vi "Wait on CMD Task.vi"(8 "error in (no error)":errorcluster, 9 "Programmer Name":string, 10 "Flash Timeout (ms)":i32=45000, 11 "Slide in":refnum<vi>) -> (0 "error out":errorcluster, 3 "Timed out?":bool)   [LabVIEW 2015]
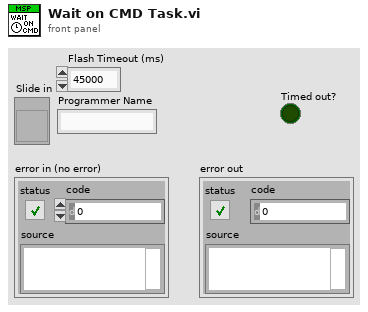
[diagram p1: front panel]
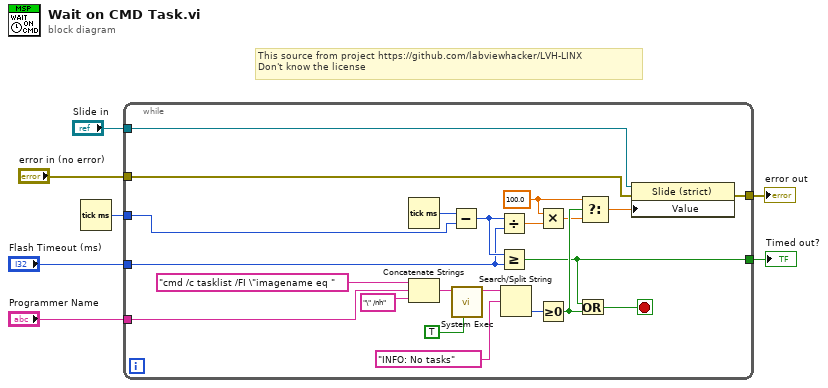
[diagram p0: block diagram]
diagram:
  # "This source from project https://github.com/labviewhacker/LVH-LINX\nDon't know the license"
  n1 = Tick Count (ms)() -> (millisecond timer value=w2:u32)
  n2 = while {
    tunnel: w2 -> [w28]
    tunnel: [w27] -> w4
    tunnel: "error in (no error)" -> [w26]
    tunnel: "Slide in" -> [w25]
    tunnel: [w13] -> w1
    tunnel: "Programmer Name" -> [w9]
    tunnel: "Flash Timeout (ms)" -> [w8]
    stop <- w19 stop-if-true
    w16 = 100.0 ("x")
    n3 = Tick Count (ms)() -> (millisecond timer value=w29:u32)
    n4 = Concatenate Strings("cmd /c tasklist /FI \"imagename eq " ("command line"), w9, "\" /nh" ("string")) -> (w11:string)
    n5 = Subtract(x=w29, y=w28) -> (x-y=w24:u32)
    n6 = call <vilib>:"System Exec.vi"("run minimized? (F)"=TRUE, "command line"=w11) -> ("standard output"=w21:string)  [unwired: 6 in, 3 out]
    n7 = Divide(x=w24, y=w8) -> (x/y=w23:dbl)
    n8 = Greater Or Equal?(x=w24, y=w8) -> (x >= y?=w13:bool)
    n9 = Search/Split String(string=w21, search string/char (-)="INFO: No tasks") -> (offset of match=w18:i32)  [unwired: 1 in, 2 out]
    n10 = Multiply(x=w16, y=w23) -> (x*y=w15:dbl)
    n11 = Greater Or Equal To 0?(x=w18) -> (x >= 0?=w17:bool)
    n12 = Or(x=w13, y=w17) -> (x .or. y?=w19:bool)
    n13 = Select(t=w16, s=w17, f=w15) -> (s? t:f=w14:dbl)
    n14 = property class="Slide (strict)"(reference=w25, error in=w26, "Value"=w14) -> (error out=w27:errorcluster)  [unwired: 1 out]
  }
  "error out" <- w4
  "Timed out?" <- w1
